vi "Auto-Stretch.vi"(4 "Vertical Padding":i16, 6 "Horizontal Padding":i16, 8 "Error In":errorcluster, 9 "Vertical?":bool=TRUE, 10 "Horizontal?":bool=TRUE) -> (0 "Error Out":errorcluster, 3 "Auto-Stretch Out":refnum<class "Auto-Stretch.lvclass">)   [LabVIEW 2020, in "Panel.lvlib" / "Auto-Stretch.lvclass"]
doc: "Calculates the size based on the visible controls and decorations on the front panel.\n\nThis will only stretch the right side and bottom of the panel to fit the farthest right and farthest down control.\n\nThis is useful when programatically positioning controls before the panel is shown to the user.\n\n<B>Horizontal:</B> Defines if the panel should stretch horizontally.\n<B>Vertical:</B> Defines if the panel should stretch vertically.\n<B>Horizontal Padding:</B> Defines the horizontal padding.\n<B>Vertical Padding:</B> Defines the vertical padding.\n<B>Error In:</B> Describes error conditions that occur before this node runs.\n\n<B>Auto-Stretch Out:</B> Auto-Stretch object.\n<B>Error Out:</B> Contains error information.\n\n----\nPlease see the following web address for additional documentation and tutorial information:\nhttp://www.mooregoodideas.com/mgi-panel-manager/\n\nAuthor: Derek Trepanier\n\nCopyright (c) 2018, Moore Good Ideas, Inc.\n\nAll rights reserved.\n\nRedistribution and use in source and binary forms, with or without modification, are permitted provided that the following conditions are met:\n\n * Redistributions of source code must retain the above copyright notice, this list of conditions and the following disclaimer.\n * Redistributions in binary form must reproduce the above copyright notice, this list of conditions and the following disclaimer in the documentation and/or other materials provided with the distribution.\n * Neither the name of Moore Good Ideas, Inc. nor the names of its contributors may be used to endorse or promote products derived from this software without specific prior written permission.\n\nTHIS SOFTWARE IS PROVIDED BY THE COPYRIGHT HOLDERS AND CONTRIBUTORS \"AS IS\" AND ANY EXPRESS OR IMPLIED WARRANTIES, INCLUDING, BUT NOT LIMITED TO, THE IMPLIED WARRANTIES OF MERCHANTABILITY AND FITNESS FOR A PARTICULAR PURPOSE ARE DISCLAIMED. IN NO EVENT SHALL THE COPYRIGHT OWNER OR CONTRIBUTORS BE LIABLE FOR ANY DIRECT, INDIRECT, INCIDENTAL, SPECIAL, EXEMPLARY, OR CONSEQUENTIAL DAMAGES (INCLUDING, BUT NOT LIMITED TO, PROCUREMENT OF SUBSTITUTE GOODS OR SERVICES; LOSS OF USE, DATA, OR PROFITS; OR BUSINESS INTERRUPTION) HOWEVER CAUSED AND ON ANY THEORY OF LIABILITY, WHETHER IN CONTRACT, STRICT LIABILITY, OR TORT (INCLUDING NEGLIGENCE OR OTHERWISE) ARISING IN ANY WAY OUT OF THE USE OF THIS SOFTWARE, EVEN IF ADVISED OF THE POSSIBILITY OF SUCH DAMAGE."
uses:
  <vilib>/MGI/Panel Manager/Panel/Window Position/Reference Position/Size/Auto-Stretch/Auto-Stretch.lvclass
  <vilib>/MGI/Panel Manager/Panel/Window Position/Reference Position/Size/Auto-Stretch/Auto-Stretch.lvclass/Auto-Stretch.ctl
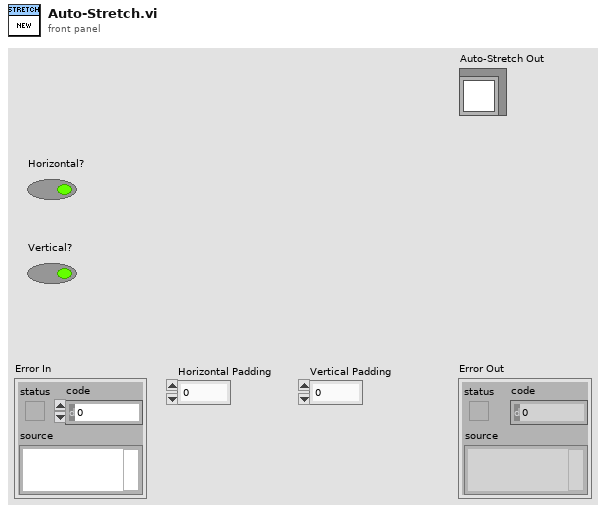
[diagram p1: front panel]
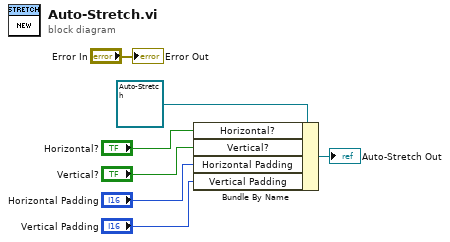
[diagram p0: block diagram]
diagram:
  n1 = Bundle By Name(cluster=refnum<class "Auto-Stretch.lvclass"> refnum ("Auto-Stretch in"), "Horizontal?"="Horizontal?", "Vertical?"="Vertical?", "Horizontal Padding"="Horizontal Padding", "Vertical Padding"="Vertical Padding") -> (→"Auto-Stretch Out":refnum<class "Auto-Stretch.lvclass">)
  "Error Out" <- "Error In"
